vi "Compare Calls.vi"(8 "error in (no error)":errorcluster, 9 "VI Call 2":refnum<class "VI Call.lvclass">, 10 "VI Call 1":refnum<class "VI Call.lvclass">, 11 "Tolerant Numeric Comparator In":refnum<class "Tolerant Numeric Argument Comparator.lvclass">) -> (0 "error out":errorcluster, 1 "Description":string, 2 "Equal?":bool)   [LabVIEW 2020, in "Tolerant Numeric Argument Comparator.lvclass"]
uses:
  Tolerant Numeric Argument Comparator.lvclass
  Core/VI Call/VI Call.lvclass
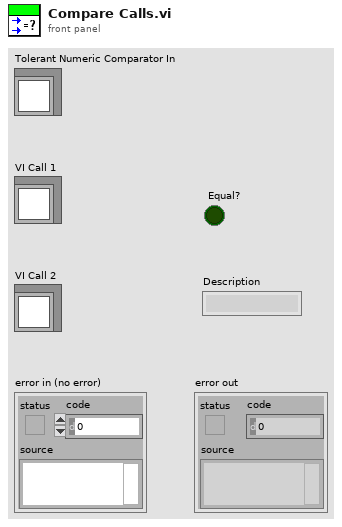
[diagram p1: front panel]
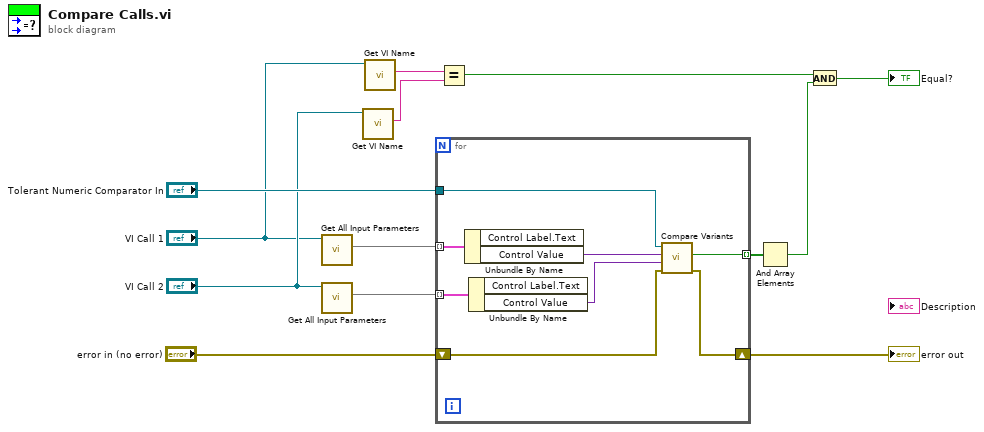
[diagram p0: block diagram]
diagram:
  n1 = call-dynamic "Get All Input Parameters.vi"("VI Call in"="VI Call 1") -> ("Input Parameters"=w13:map{string, variant})  [unwired: 9 in, 1 out]
  n2 = call-dynamic "Get All Input Parameters.vi"("VI Call in"="VI Call 2") -> ("Input Parameters"=w12:map{string, variant})  [unwired: 9 in, 1 out]
  n3 = call-dynamic "Get VI Name.vi"("VI Call In"="VI Call 2") -> ("VI Name"=w1:string)  [unwired: 9 in, 1 out]
  n4 = call-dynamic "Get VI Name.vi"("VI Call In"="VI Call 1") -> ("VI Name"=w2:string)  [unwired: 9 in, 1 out]
  n5 = for {
    tunnel: w13 -> [w21] mode=indexing
    tunnel: w12 -> [w20] mode=indexing
    tunnel: "Tolerant Numeric Comparator In" -> [w17]
    tunnel: [w16] -> w10 mode=indexing
    shift-right: [w14] -> w8
    shift-left: "error in (no error)" -> [w15]
    n6 = Unbundle By Name(w21) -> ("Control Value"=w19:variant)  [unwired: 1 out]
    n7 = Unbundle By Name(w20) -> ("Control Value"=w18:variant)  [unwired: 1 out]
    n8 = call "Compare Variants.vi"("error in (no error)"=w15, "Variant 2"=w18, "Variant 1"=w19, "Tolerant Numeric Comparator In"=w17) -> ("error out"=w14:errorcluster, "Equal?"=w16:bool)  [unwired: 5 in, 1 out]
  }
  "error out" <- w8
  n9 = Equal?(x=w2, y=w1) -> (x = y?=w7:bool)
  n10 = And Array Elements(Boolean array=w10) -> (logical AND=w4:bool)
  n11 = And(x=w7, y=w4) -> (x .and. y?=→"Equal?":bool)
